vi "Z900_navX_RefNum_GetSet.vi"(8 "error in (no error)":errorcluster, 9 "menu":enum16{"set", "get", "delete"}(ring), 10 "refnum name":string, 11 "navX Device":T1={"Interface"={"Protocol"=enum."SERIAL", "Update Rate (4Hz-100Hz)"=4, "navX Open TypeDef"=variant}, "Notify Packet"=refnum, "Loop VI Refnum"=refnum, "Ready to Close Occurrence Refnum"=refnum} {"Interface"."Update Rate (4Hz-100Hz)" min=4 max=60 step=1}) -> (0 "error out":errorcluster, 3 "navX Device":T1={"Interface"={"Protocol"=enum."SERIAL", "Update Rate (4Hz-100Hz)"=4, "navX Open TypeDef"=variant}, "Notify Packet"=refnum, "Loop VI Refnum"=refnum, "Ready to Close Occurrence Refnum"=refnum} {"Interface"."Update Rate (4Hz-100Hz)" min=4 max=60 step=1})   [LabVIEW 2015, in "navX Library v2.lvlib"]
doc: "Sets a reference into a registry, gets a reference from a registry, or deletes a reference from a registry. The reference is accessed by name, and can be given any unique name."
uses:
  navX Library v2.lvlib
  TypeDefs/Z900_navX_DeviceTypeDef.ctl
  TypeDefs/Z900_navX_ProtocolTypeDef.ctl
  TypeDefs/Z900_navX_NotifyPacketTypeDef.ctl
  TypeDefs/Z900_navX_ActionTypeDef.ctl
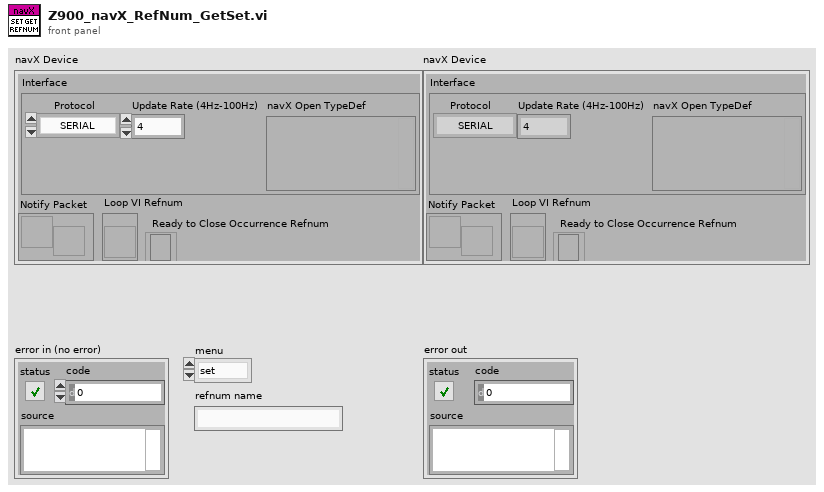
[diagram p1: front panel]
types:
  T1 = typedef "navX Library v2.lvlib/Z900_navX_DeviceTypeDef.ctl" = cluster{"Interface":cluster{"Protocol":T2, "Update Rate (4Hz-100Hz)":u8, "navX Open TypeDef":variant}, "Notify Packet":refnum<notifier>, "Loop VI Refnum":refnum<vi>, "Ready to Close Occurrence Refnum":refnum<k4>}
  T2 = typedef "navX Library v2.lvlib/Z900_navX_ProtocolTypeDef.ctl" = enum16{"SERIAL", "I2C", "SPI"}
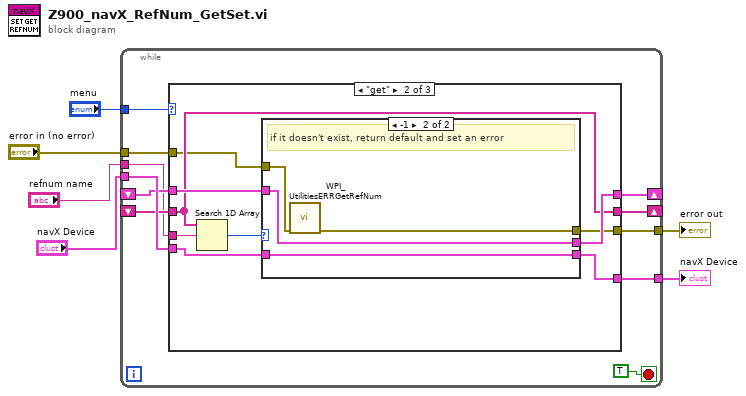
[diagram p0: block diagram]
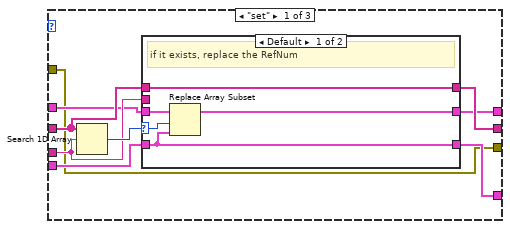
[diagram p2: hidden frame]
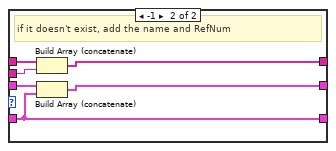
[diagram p3: hidden frame]
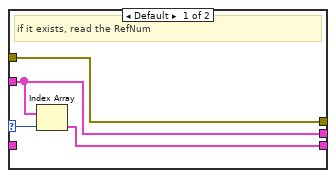
[diagram p4: hidden frame]
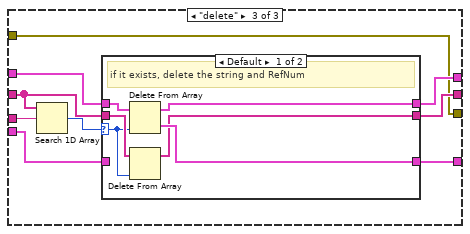
[diagram p5: hidden frame]
diagram:
  n1 = while {
    tunnel: "navX Device" -> [w17]
    tunnel: "refnum name" -> [w10]
    tunnel: "error in (no error)" -> [w9]
    shift-right: [w16] -> _
    shift-left: _ -> [w15]
    tunnel: [w14] -> w1
    tunnel: "menu" -> [w13]
    shift-right: [w12] -> _
    shift-left: _ -> [w11]
    tunnel: [w8] -> w3
    stop <- TRUE stop-if-true
    n2 = case shown="\"get\"" w13 {
      tunnel: w17 -> [w21 w43 w58]
      tunnel: [w20 w42 w57] -> w16
      tunnel: w15 -> [w22 w44 w59]
      tunnel: [w19 w41 w56] -> w14
      tunnel: [w26 w40 w63] -> w12
      tunnel: w11 -> [w25 w40 w62]
      tunnel: w10 -> [w23 w45 w60]
      tunnel: [w18 w38 w55] -> w8
      tunnel: w9 -> [w18 w39 w55]
      frame "set" {
        n3 = Search 1D Array(1D array=w25, element=w23) -> (index of element=w24:i32)  [unwired: 1 out]
        n4 = case shown="Default" w24 {
          selector: w24 -> [w29 _]
          tunnel: [w31 w37] -> w26
          tunnel: w25 -> [w31 w36]
          tunnel: w23 -> [_ w35]
          tunnel: w22 -> [w30 w34]
          tunnel: w21 -> [w27 w32]
          tunnel: [w28 w33] -> w20
          tunnel: [w27 w32] -> w19
          frame Default {
            # "if it exists, replace the RefNum"
            n5 = Replace Array Subset(array=w30, new element=w27, index=w29) -> (w28:T1[])
          }
          frame -1 {
            # "if it doesn't exist, add the name and RefNum"
            n6 = Build Array (concatenate)(w36, w35) -> (w37:string[])
            n7 = Build Array (concatenate)(w34, w32) -> (w33:T1[])
          }
        }
      }
      frame "get" {
        n8 = Search 1D Array(1D array=w40, element=w45) -> (index of element=w46:i32)  [unwired: 1 out]
        n9 = case shown="-1" w46 {
          selector: w46 -> [w50 _]
          tunnel: w44 -> [w48 w54]
          tunnel: w43 -> [_ w51]
          tunnel: [w48 w54] -> w42
          tunnel: [w49 w51] -> w41
          tunnel: w39 -> [w47 w53]
          tunnel: [w47 w52] -> w38
          frame Default {
            # "if it exists, read the RefNum"
            n10 = Index Array(array=w48, index=w50) -> (element=w49:T1)
          }
          frame -1 {
            # "if it doesn't exist, return default and set an error"
            n11 = call <vilib>:"WPI_UtilitiesERRGetRefNum.vi"("error in (no error)"=w53) -> ("ERRGetRefNum"=w52:errorcluster)  [unwired: 10 out]
          }
        }
      }
      frame "delete" {
        n12 = Search 1D Array(1D array=w62, element=w60) -> (index of element=w61:i32)  [unwired: 1 out]
        n13 = case shown="Default" w61 {
          selector: w61 -> [w64 _]
          tunnel: [w65 w71] -> w63
          tunnel: w62 -> [w66 w71]
          tunnel: w59 -> [w69 w70]
          tunnel: w58 -> [_ w72]
          tunnel: [w68 w70] -> w57
          tunnel: [w67 w72] -> w56
          frame Default {
            # "if it exists, delete the string and RefNum"
            n14 = Delete From Array(array=w69, index=w64) -> (deleted portion=w67:T1, array with subset deleted=w68:T1[])  [unwired: 1 in]
            n15 = Delete From Array(array=w66, index=w64) -> (array with subset deleted=w65:string[])  [unwired: 1 in, 1 out]
          }
          frame -1 {
            # "if it doesn't exist, do nothing"
          }
        }
      }
    }
  }
  "navX Device" <- w1
  "error out" <- w3
